vi "Write BallOutOfFieldPlay.vi"(8 "error in (no error)":errorcluster, 10 "BallOutOfFieldPlay":refnum<class "BallOutOfFieldPlay.lvclass">, 11 "Playbook in":refnum<class "Playbook.lvclass">) -> (0 "error out":errorcluster, 3 "Playbook out":refnum<class "Playbook.lvclass">)   [LabVIEW 2018, in "Playbook.lvclass"]
uses:
  Playbook.lvclass
  BallOutOfFieldPlay_class/BallOutOfFieldPlay.lvclass
  Playbook.lvclass/Playbook.ctl
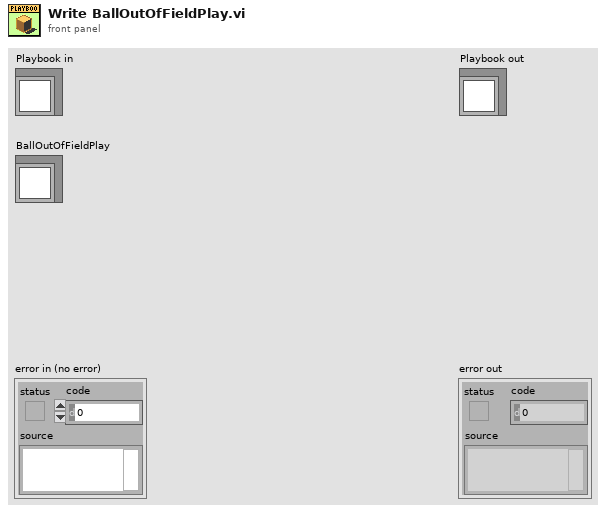
[diagram p1: front panel]
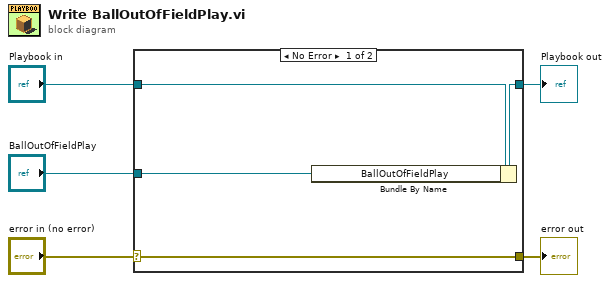
[diagram p0: block diagram]
diagram:
  n1 = case shown="No Error" "error in (no error)" {
    selector: "error in (no error)" -> [w9 w10]
    tunnel: [w9 w10] -> w4
    tunnel: [w7 w11] -> w2
    tunnel: "Playbook in" -> [w8 w11]
    tunnel: "BallOutOfFieldPlay" -> [w6 _]
    frame No Error {
      n2 = Bundle By Name(cluster=w8, "BallOutOfFieldPlay"=w6) -> (w7:refnum<class "Playbook.lvclass">)
    }
    frame Error {
    }
  }
  "error out" <- w4
  "Playbook out" <- w2
